vi "GeraSinalSenoide.vi"(0 "params":variant, 2 "Tx Aquisicao":dbl, 4 "estadoIn":variant) -> (15 "sinal":waveform(dbl), 18 "estadoOut":variant)   [LabVIEW 2017]
uses:
  Typedefs/Tipo_ParamsSenoide.ctl
  <vilib>/Analysis/NI_AALBase.lvlib
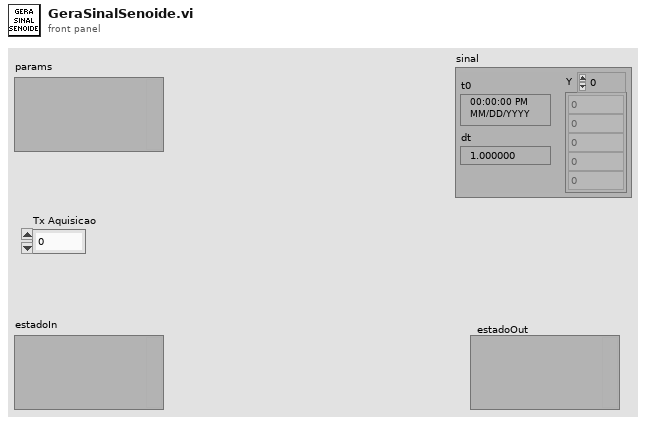
[diagram p1: front panel]
types:
  T1 = typedef "Tipo_ParamsSenoide.ctl" = cluster{"Amplitude":dbl, "Frequencia":dbl, "Fase":dbl}
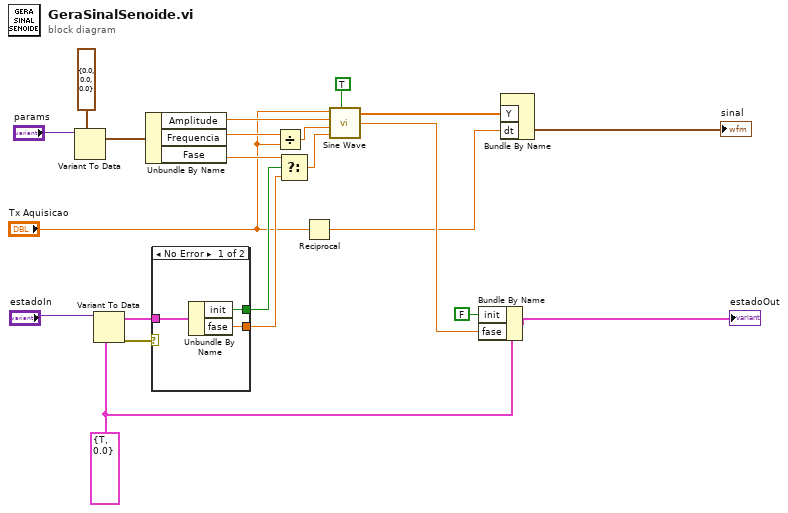
[diagram p0: block diagram]
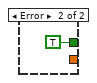
[diagram p2: hidden frame]
diagram:
  w9 = cluster{"init":bool, "fase":dbl} {"init"=TRUE, "fase"=0.0}
  n1 = Variant To Data(type=T1 {"Amplitude"=0.0, "Frequencia"=0.0, "Fase"=0.0} ("Tipo_ParamSenoide"), Variant="params") -> (data=w20:T1)  [unwired: 1 in, 1 out]
  n2 = Variant To Data(type=w9, Variant="estadoIn") -> (data=w16:cluster{"init":bool, "fase":dbl}, error out=w10:errorcluster)  [unwired: 1 in]
  n3 = Unbundle By Name(w20) -> ("Amplitude"=w19:dbl, "Frequencia"=w2:dbl, "Fase"=w15:dbl)
  n4 = case shown="No Error" w10 {
    tunnel: w16 -> [w25 _]
    tunnel: [w24 TRUE ("init")] -> w14
    tunnel: [w23 _] -> w11
    frame No Error {
      n5 = Unbundle By Name(w25) -> ("init"=w24:bool, "fase"=w23:dbl)
    }
    frame Error {
    }
  }
  n6 = Divide(x=w2, y="Tx Aquisicao") -> (x/y=w18:dbl)
  n7 = Select(t=w15, s=w14, f=w11) -> (s? t:f=w13:dbl)
  n8 = Reciprocal(x="Tx Aquisicao") -> (1/x=w4:dbl)
  n9 = call <vilib>:"Sine Wave.vi"("samples"="Tx Aquisicao", "amplitude"=w19, "frequency"=w18, "phase in"=w13, "reset phase"=TRUE) -> ("sine wave"=w5:dbl[], "phase out"=w6:dbl)  [unwired: 1 out]
  n10 = Bundle By Name(cluster=w9, "init"=FALSE, "fase"=w6) -> (→"estadoOut":cluster{"init":bool, "fase":dbl})
  n11 = Bundle By Name("Y"=w5, "dt"=w4) -> (→"sinal":waveform(dbl))  [unwired: 1 in]
